vi "Pixel_Index_to_Wavelength.vi"(3 "pixel index":dbl=512.0 min=0.0 max=1024.0 format="%.2f", 4 "File Info In":T1={"FilePath"=path "/Volumes/DATA/Labview Items", "Field (T)"=12.0, "Temperature (K)"=12.0, "X-Axis"=enum."nm", "Center nm"=-1.0, "Current Grating Density"=enum."600", "CCD Parameters"={"Exposure Time (s)"=0.2, "Offset"=0.0, "BkgrdCrct"=FALSE, "Shutter"=FALSE, "Mode"=enum."Regular", "Repetition"=4, "dt or s"=0.0}, "Operation Mode"=enum."NML Data Acquisition", "Exp Index"=3, "Index_repetition"=0, "Index"=0, "Current Detector"=enum."CCD-1024x256"} {"CCD Parameters"."dt or s" format="%#.6f"; "CCD Parameters"."Repetition" min=1; "CCD Parameters"."Offset" format="%#.2f"; "CCD Parameters"."Exposure Time (s)" min=0.02 max=6000.0 format="%#.2f"; "Center nm" format="%.2f"; "Temperature (K)" format="%.2f"; "Field (T)" format="%.2f"}, 5 "Central Wavelength":dbl=600.0 format="%.2f") -> (1 "nm (out)":dbl=571.2504622529284 format="%.4f")   [LabVIEW 2025]
doc: "Author: Scott Hannahs <sth@magnet.fsu.edu>\n\nThis software is licensed for use under the “MIT License\"\nCopyright (c) 2025 Scott Hannahs, sth@sth@magnet.sthnet.net\n\nPermission is hereby granted, free of charge, to any person obtaining a copy of this software and associated documentation files (the \"Software\"), to deal in the Software without restriction, including without limitation the rights to use, copy, modify, merge, publish, distribute, sublicense, and/or sell copies of the Software, and to permit persons to whom the Software is furnished to do so, subject to the following conditions: The above copyright notice and this permission notice shall be included in all copies or substantial portions of the Software.\n\nTHE SOFTWARE IS PROVIDED \"AS IS\", WITHOUT WARRANTY OF ANY KIND, EXPRESS OR IMPLIED, INCLUDING BUT NOT LIMITED TO THE WARRANTIES OF MERCHANTABILITY, FITNESS FOR A PARTICULAR PURPOSE AND NONINFRINGEMENT. IN NO EVENT SHALL THE AUTHORS OR COPYRIGHT HOLDERS BE LIABLE FOR ANY CLAIM, DAMAGES OR OTHER LIABILITY, WHETHER IN AN ACTION OF CONTRACT, TORT OR OTHERWISE, ARISING FROM, OUT OF OR IN CONNECTION WITH THE SOFTWARE OR THE USE OR OTHER DEALINGS IN THE SOFTWARE."
uses:
  Globals and TypeDefs/Type Definitions.llb/FileInfoParameter.ctt
  Globals and TypeDefs/Type Definitions.llb/Wavelength Unit.ctt
  Globals and TypeDefs/Type Definitions.llb/McPherson Grating Density.ctl
  Globals and TypeDefs/Type Definitions.llb/CCDParameter.ctt
  Globals and TypeDefs/Type Definitions.llb/OperationMode.ctt
  Globals and TypeDefs/Type Definitions.llb/ListOfDetectors.ctt
panel:
  out "Detector Pixel Distance":dbl=27.0 format="%.2f"
  out "beta":dbl=0.03851514953863218 format="%.2f"
  out "alpha":dbl=21.141484850461367 format="%.2f"
  out "Spectrometer Mirror angle":dbl=21.18 format="%.2f"
  out "Spectrometer Focal length":dbl=750.0 format="%.1f"
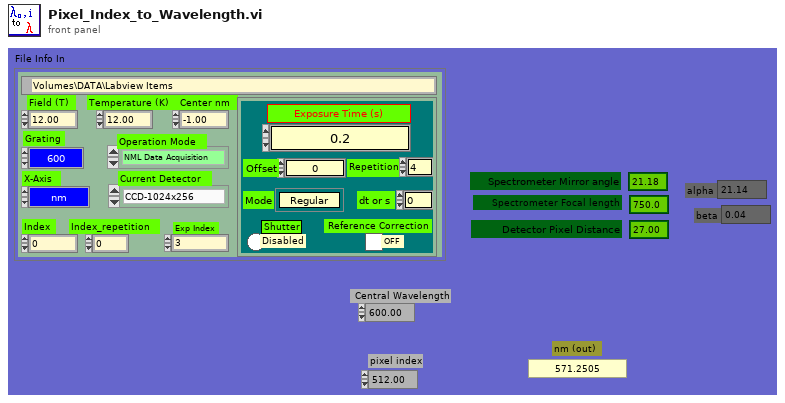
[diagram p1: front panel]
types:
  T1 = typedef "FileInfoParameter.ctt" = cluster{"FilePath":path, "Field (T)":dbl, "Temperature (K)":dbl, "X-Axis":T2, "Center nm":dbl, "Current Grating Density":T3, "CCD Parameters":T4, "Operation Mode":T5, "Exp Index":u32, "Index_repetition":u16, "Index":u16, "Current Detector":T6}
  T2 = typedef "Wavelength Unit.ctt" = enum8{"Point", "nm", "eV", "meV", "cm_1"}
  T3 = typedef "McPherson Grating Density.ctl" = enum8{"150", "300", "600", "1200", "1800"}
  T4 = typedef "CCDParameter.ctt" = cluster{"Exposure Time (s)":dbl, "Offset":dbl, "BkgrdCrct":bool, "Shutter":bool, "Mode":enum8{"Regular", "OverExp Cor", "SpikeRemove", "ForCalibration"}, "Repetition":u16, "dt or s":dbl}
  T5 = typedef "OperationMode.ctt" = enum16{"Standby", "CCD Single Shot", "CCD Sequence Shots", "CCD Custom Shots", "CCD Reference Shot", "Step Scanning ", "Time Scanning", "NML Data Acquisition"}
  T6 = typedef "ListOfDetectors.ctt" = enum8{"CCD-1024x256", "InGaAs PDA-1024x1", "CCD-1340x400", "Ge Single Channel", "Si Single Channel", "PMT Single Channel"}
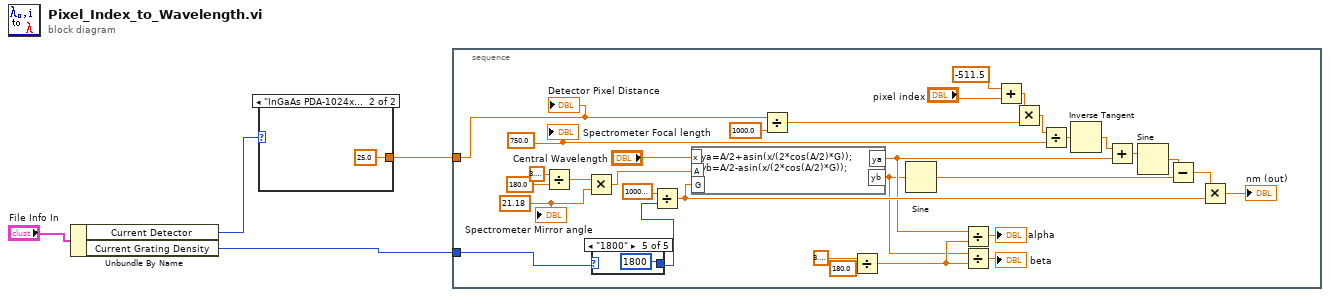
[diagram p0: block diagram]
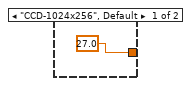
[diagram p2: hidden frame]
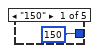
[diagram p3: hidden frame]
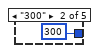
[diagram p4: hidden frame]
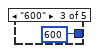
[diagram p5: hidden frame]
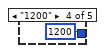
[diagram p6: hidden frame]
diagram:
  n1 = Unbundle By Name("File Info In") -> ("Current Detector"=w4:T6, "Current Grating Density"=w1:T3)
  n2 = case shown="\"InGaAs PDA-1024x1\"" w4 {
    tunnel: [27.0 ("x") 25.0 ("x")] -> w3
    frame "CCD-1024x256", Default {
    }
    frame "InGaAs PDA-1024x1" {
    }
  }
  n3 = stacked-sequence {
    tunnel: w3 -> [w8]
    tunnel: w1 -> [w7]
    frame #0 {
      w32 = 21.18 ("Detector Pixel Distance")
      w31 = 750.0 ("Detector Pixel Distance")
      n4 = Divide(x=3.141592653589793, y=180.0) -> (x/y=w25:dbl)
      n5 = Multiply(x=w25, y=w32) -> (x*y=w30:dbl)
      n6 = case shown="\"1800\"" w7 {
        tunnel: [150 300 600 1200 1800] -> w20
        frame "150" {
        }
        frame "300" {
        }
        frame "600" {
        }
        frame "1200" {
        }
        frame "1800" {
        }
      }
      n7 = Divide(x=1000000.0, y=w20) -> (x/y=w29:dbl)
      n8 = formula code="ya=A/2+asin(x/(2*cos(A/2)*G));\nyb=A/2-asin(x/(2*cos(A/2)*G));"("x"="Central Wavelength", "A"=w30, "G"=w29) -> ("ya"=w23:dbl, "yb"=w22:dbl)
      n9 = Divide(x=w8, y=1000.0) -> (x/y=w34:dbl)
      n10 = Divide(x=3.141592653589793, y=180.0) -> (x/y=w28:dbl)
      n11 = Sine(x=w22) -> (sin(x)=w33:dbl)
      n12 = Divide(x=w23, y=w28) -> (x/y=→"alpha":dbl)
      n13 = Divide(x=w22, y=w28) -> (x/y=→"beta":dbl)
      n14 = Add(x=-511.5, y="pixel index") -> (x+y=w11:dbl)
      n15 = Multiply(x=w11, y=w34) -> (x*y=w13:dbl)
      n16 = Divide(x=w13, y=w31) -> (x/y=w16:dbl)
      n17 = Inverse Tangent(1:w16) -> (0:w15:dbl)
      n18 = Add(x=w15, y=w23) -> (x+y=w14:dbl)
      n19 = Sine(x=w14) -> (sin(x)=w18:dbl)
      n20 = Subtract(x=w18, y=w33) -> (x-y=w17:dbl)
      n21 = Multiply(x=w17, y=w29) -> (x*y=→"nm (out)":dbl)
      "Spectrometer Focal length" <- w31
      "Spectrometer Mirror angle" <- w32
      "Detector Pixel Distance" <- w8
    }
  }
